vi "Wait for Aircraft Heartbeat.vi"(8 "error out":errorcluster, 11 "Aircraft COM Port":refnum<visa-resource-name>) -> (0 "error out 2":errorcluster, 1 "Aircraft ID":u8, 2 "Message Complete":bool, 3 "Aircraft COM Port 2":refnum<visa-resource-name>)   [LabVIEW 2014]
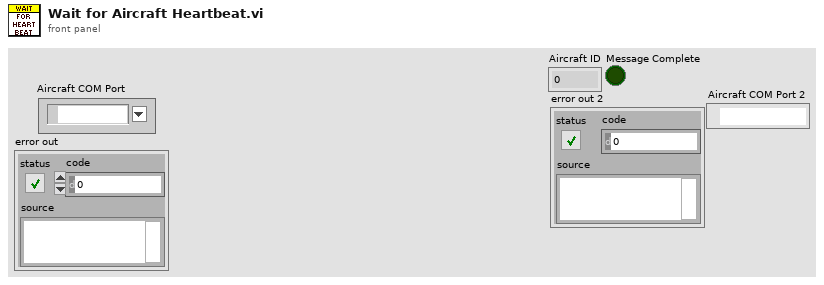
[diagram p1: front panel]
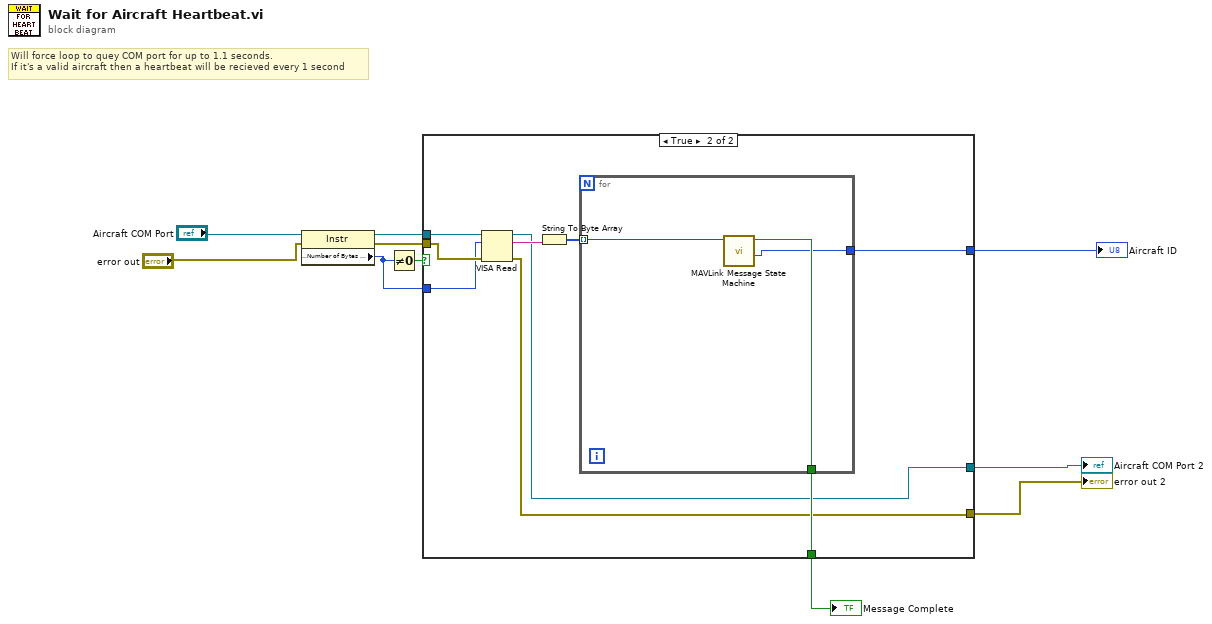
[diagram p0: block diagram]
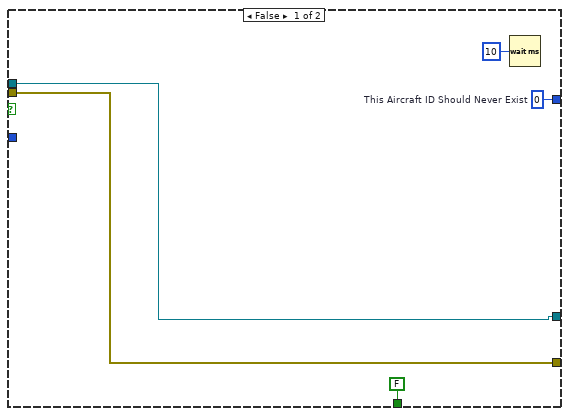
[diagram p2: hidden frame]
diagram:
  # "Will force loop to quey COM port for up to 1.1 seconds.\nIf it's a valid aircraft then a heartbeat will be recieved every 1 second"
  n1 = property class="Instr"(reference="Aircraft COM Port", error in="error out") -> (reference out=w5:refnum<visa-resource-name>, error out=w4:errorcluster, "Serial Settings:Number of Bytes at Serial Port"=w3:u32)
  n2 = Not Equal To 0?(x=w3) -> (x != 0?=w6:bool)
  n3 = case shown="True" w6 {
    tunnel: w5 -> [w12 w24]
    tunnel: w4 -> [w13 w23]
    tunnel: w3 -> [_ w22]
    tunnel: [FALSE ("Message Complete") w19] -> w2
    tunnel: [w14 w18] -> w9
    tunnel: [w13 w17] -> w8
    tunnel: [w12 w16] -> w7
    frame False {
      w14 = u8 0  # This Aircraft ID Should Never Exist
      n4 = Wait (ms)(milliseconds to wait=u32 10) -> ()  [unwired: 1 out]
    }
    frame True {
      n5 = VISA Read(VISA resource name=w24, byte count=w22, error in (no error)=w23) -> (VISA resource name out=w16:refnum<visa-resource-name>, read buffer=w21:string, error out=w17:errorcluster)  [unwired: 1 out]
      n6 = String To Byte Array(string=w21) -> (unsigned byte array=w20:u8[])
      n7 = for {
        tunnel: w20 -> [w27] mode=indexing
        tunnel: [w26] -> w19
        tunnel: [w25] -> w18
        n8 = call "MAVLink Message State Machine.vi"("Incoming Bytes"=w27) -> ("Aircraft ID"=w25:u8, "Message Complete"=w26:bool)  [unwired: 8 in, 1 out]
      }
    }
  }
  "Aircraft ID" <- w9
  "error out 2" <- w8
  "Aircraft COM Port 2" <- w7
  "Message Complete" <- w2
